vi "Set Voltage of PS1.vi"(8 "error in (no error)":errorcluster, 9 "Current Limit (0)":dbl min=0.0 max=6.0 format="%#.2g", 10 "Output Voltage (0)":dbl min=0.0 max=18.0 format="%#.2f", 11 "PS 1":refnum<visa-resource-name>) -> (0 "error out":errorcluster)   [LabVIEW 2015]
uses:
  <instrlib>/BK Precision 178XB Series/BK Precision 178XB Series.lvlib
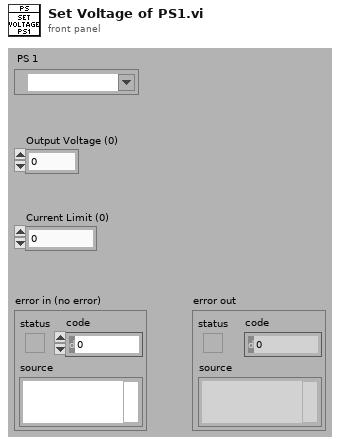
[diagram p1: front panel]
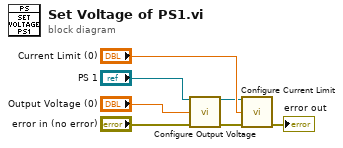
[diagram p0: block diagram]
diagram:
  n1 = call <instrlib>:"Configure Output Voltage.vi"("VISA resource name"="PS 1", "Output Voltage (0)"="Output Voltage (0)", "error in (no error)"="error in (no error)") -> ("VISA resource name out"=w2:refnum<visa-resource-name>, "error out"=w3:errorcluster)  [unwired: 11 in]
  n2 = call <instrlib>:"Configure Current Limit.vi"("VISA resource name"=w2, "Current Limit (0)"="Current Limit (0)", "error in (no error)"=w3) -> ("error out"=→"error out":errorcluster)  [unwired: 11 in, 1 out]
